vi "Execution_Message_BuildLogMessage.vi"(8 "error in":errorcluster, 11 "ErrorMessage in":refnum<class "ErrorMessage.lvclass">) -> (0 "error out":errorcluster, 3 "ErrorMessage out":refnum<class "ErrorMessage.lvclass">)   [LabVIEW 2013, in "ErrorMessage.lvclass"]
uses:
  ErrorMessage.lvclass
  Messages.lvclass
  ErrorMessage.lvclass/ErrorMessage.ctl
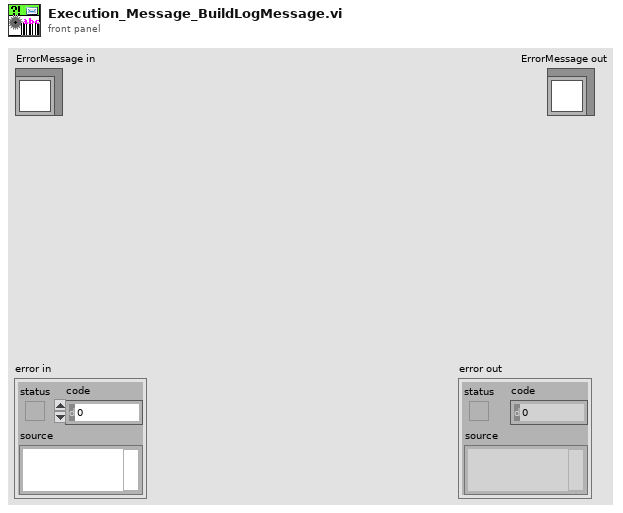
[diagram p1: front panel]
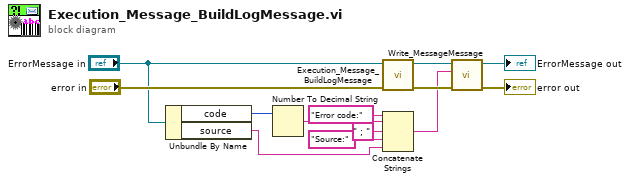
[diagram p0: block diagram]
diagram:
  n1 = Unbundle By Name("ErrorMessage in") -> ("code"=w11:i32, "source"=w6:string)
  n2 = Number To Decimal String(number=w11) -> (decimal integer string=w10:string)  [unwired: 1 in]
  n3 = call-parent "Execution_Message_BuildLogMessage.vi"("error in (no error)"="error in", "Messages in"="ErrorMessage in") -> ("error out"=w3:errorcluster, "Messages out"=w5:refnum<class "ErrorMessage.lvclass">)  [unwired: 8 in]
  n4 = Concatenate Strings("Error code:" ("string"), w10, " ; " ("string"), "Source:" ("string"), w6) -> (w1:string)
  n5 = call-dynamic "Write_MessageMessage.vi"("error in (no error)"=w3, "Message"=w1, "Messages in"=w5) -> ("error out"=→"error out":errorcluster, "Messages out"=→"ErrorMessage out":refnum<class "ErrorMessage.lvclass">)  [unwired: 7 in]
